vi "Read Default Core.vi"(8 "error in (no error)":errorcluster, 9 "Name":string, 10 "Path":path, 11 "Cluster In":variant) -> (0 "error out":errorcluster, 3 "Cluster Out":variant)   [LabVIEW 2019, in "ObjectSettings.lvclass"]
uses:
  ObjectSettings.lvclass
  <userlib>/LevyLab/Configuration/Configuration.lvclass
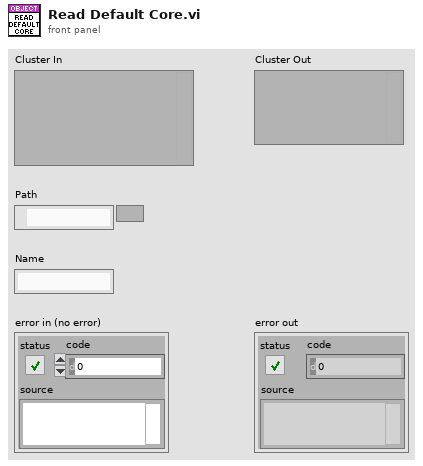
[diagram p1: front panel]
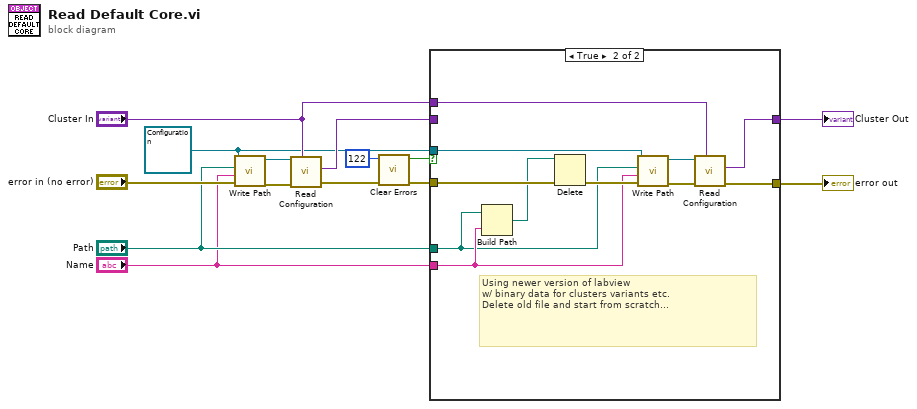
[diagram p0: block diagram]
diagram:
  w3 = refnum<class "Configuration.lvclass"> refnum ("Configuration in")
  n1 = call <userlib>:"Write Path.vi"("error in (no error)"="error in (no error)", "Filename [Configuration.ini]"="Name", "Path"="Path", "Configuration in"=w3) -> ("error out"=w12:errorcluster, "Configuration out"=w13:refnum<class "Configuration.lvclass">)  [unwired: 6 in]
  n2 = call <userlib>:"Read Configuration.vi"("INI Fomatted Cluster Type"="Cluster In", "error in (no error)"=w12, "Configuration in"=w13) -> ("error out"=w10:errorcluster, "Configuration"=w5:variant)  [unwired: 6 in, 1 out]
  n3 = call <vilib>:"Clear Errors.vi"("error in (no error)"=w10, "specific error code to clear (0: all)"=122) -> ("error out"=w9:errorcluster, "specific error cleared?"=w8:bool)  [unwired: 4 in]
  n4 = case shown="True" w8 {
    tunnel: w9 -> [w15 w27]
    tunnel: [w15 w20] -> w7
    tunnel: [w16 w21] -> w6
    tunnel: w5 -> [w16 _]
    tunnel: "Cluster In" -> [_ w22]
    tunnel: w3 -> [_ w23]
    tunnel: "Path" -> [_ w17]
    tunnel: "Name" -> [_ w19]
    frame False {
    }
    frame True {
      # "Using newer version of labview\nw/ binary data for clusters variants etc.\nDelete old file and start from scratch..."
      n5 = Build Path(base path=w17, name or relative path=w19) -> (appended path=w18:path)
      n6 = Delete(path (use dialog)=w18, error in=w27) -> (error out=w26:errorcluster)  [unwired: 3 in, 2 out]
      n7 = call <userlib>:"Write Path.vi"("error in (no error)"=w26, "Filename [Configuration.ini]"=w19, "Path"=w17, "Configuration in"=w23) -> ("error out"=w25:errorcluster, "Configuration out"=w24:refnum<class "Configuration.lvclass">)  [unwired: 6 in]
      n8 = call <userlib>:"Read Configuration.vi"("INI Fomatted Cluster Type"=w22, "error in (no error)"=w25, "Configuration in"=w24) -> ("error out"=w20:errorcluster, "Configuration"=w21:variant)  [unwired: 6 in, 1 out]
    }
  }
  "Cluster Out" <- w6
  "error out" <- w7
